vi "FileDependency.Get.Target Path.vi"(8 "error in (no error)":errorcluster, 10 "Bitfile 986x":string, 11 "Item Ref in":T1 format="%.0x") -> (0 "error out":errorcluster, 1 "Target Path":path, 2 "Source Path":path, 3 "Item Ref out":T1 format="%.0x")   [LabVIEW 2015, in "Diagnostics Addon System Explorer.lvlib"]
uses:
  Diagnostics Addon System Explorer.lvlib
  <vilib>/NI Veristand/Custom Device API/Custom Device Item Ref.ctl
  <vilib>/NI Veristand/Custom Device API/Custom Device Target Type.ctl
  <vilib>/NI Veristand/Custom Device API/Get Item Property (Dependent File).vi
  <vilib>/NI Veristand/Custom Device API/Custom Device API.lvlib
  <vilib>/NI Veristand/Custom Device Tools/Custom Device Utility Library/Custom Device Utility Library.lvlib
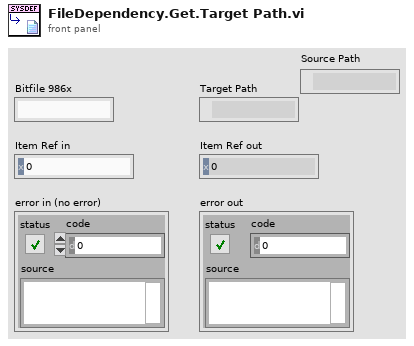
[diagram p1: front panel]
types:
  T1 = typedef "Custom Device API.lvlib/Custom Device Item Ref.ctl" = u64
  T2 = typedef "Custom Device API.lvlib/Custom Device Target Type.ctl" = enum16{"PharLap", "VxWorks", "Windows"}
  T3 = typedef "Custom Device API.lvlib/Dependent File Optional Info.ctl" = cluster{"Version":string, "RTDestination":path, "ForceDownload":bool, "SupportedTarget":string, "MD5":string}
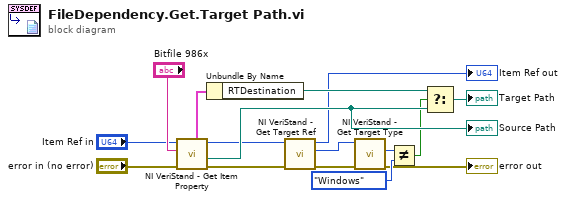
[diagram p0: block diagram]
diagram:
  n1 = call-poly <vilib>:"NI VeriStand - Get Item Property.vi"("error in (no error)"="error in (no error)", "Property Name"="Bitfile 986x", "Item Ref in"="Item Ref in") -> ("error out"=w6:errorcluster, "Path"=w16:path, "Item Ref out"=w7:T1, "OptionalInfo"=w4:T3)  [unwired: 4 in, 1 out]
  "Source Path" <- w16
  n2 = Unbundle By Name(w4) -> ("RTDestination"=w14:path)
  n3 = call <vilib>:"NI VeriStand - Get Target Ref.vi"("error in"=w6, "Item Ref in"=w7) -> ("error out"=w5:errorcluster, "Target Ref"=w8:T1, "Item Ref out"=→"Item Ref out":T1)  [unwired: 6 in, 1 out]
  n4 = call <vilib>:"NI VeriStand - Get Target Type.vi"("error in (no error)"=w5, "Item Ref in"=w8) -> ("error out"=→"error out":errorcluster, "Target Type"=w11:T2)  [unwired: 7 in, 1 out]
  n5 = Not Equal?(x=w11, y=Custom_Device_Target_Type."Windows") -> (x != y?=w13:bool)
  n6 = Select(t=w14, s=w13, f=w16) -> (s? t:f=→"Target Path":path)
